vi "Single Slow IV v1.9.vi"() -> ()   [LabVIEW 2024]
uses:
  <vilib>/Utility/file.llb/Write Delimited Spreadsheet (DBL).vi
panel:
  out "Measured current":dbl=9.843554687500001e-05
  out "Current variable":dbl=8.0
  in  "stop":bool
  in  "Tab Control 2":T1(tab)
  out "cRIO data plot":cluster{"Y":dbl[], "Y":dbl[]}[](graph)=[{"Y"=[-8.0, -7.9, -7.8, -7.7, -7.6, -7.5, -7.4, -7.3, -7.2, -7.1, -7.0, -6.9, -6.8, -6.7, -6.6, -6.5, -6.4, -6.3, -6.2, -6.1, -6.0, -5.9, -5.8, -5.699999999999999, -5.6, -5.5, -5.4, -5.3, -5.199999999999999, -5.1, -5.0, -4.9, -4.8, -4.699999999999999, -4.6, -4.5, -4.4, -4.3, -4.199999999999999, -4.1, -4.0, -3.8999999999999995, -3.8, -3.7, -3.5999999999999996, -3.5, -3.3999999999999995, -3.3, -3.1999999999999993, -3.0999999999999996, -3.0, -2.8999999999999995, -2.8, -2.6999999999999993, -2.5999999999999996, -2.5, -2.3999999999999995, -2.3, -2.1999999999999993, -2.0999999999999996, -2.0, -1.8999999999999995, -1.7999999999999998, -1.6999999999999993, -1.5999999999999996, -1.5, -1.3999999999999995, -1.2999999999999998, -1.1999999999999993, -1.0999999999999996, -1.0, -0.8999999999999995, -0.7999999999999998, -0.6999999999999993, -0.5999999999999996, -0.5, -0.39999999999999947, -0.2999999999999998, -0.1999999999999993, -0.09999999999999964, 0.0, 0.09999999999999964, 0.20000000000000107, 0.3000000000000007, 0.40000000000000036, 0.5, 0.5999999999999996, 0.7000000000000011, 0.8000000000000007, 0.9000000000000004, 1.0, 1.0999999999999996, 1.200000000000001, 1.3000000000000007, 1.4000000000000004, 1.5, 1.6000000000000014, 1.700000000000001, 1.8000000000000007, 1.9000000000000004, 2.0, 2.1000000000000014, 2.200000000000001, 2.3000000000000007, 2.4000000000000004, 2.5, 2.6000000000000014, 2.700000000000001, 2.8000000000000007, 2.9000000000000004, 3.0, 3.1000000000000014, 3.200000000000001, 3.3000000000000007, 3.4000000000000004, 3.5, 3.6000000000000014, 3.700000000000001, 3.8000000000000007, 3.9000000000000004, 4.0, 4.100000000000001, 4.200000000000001, 4.300000000000001, 4.4, 4.5, 4.600000000000001, 4.700000000000001, 4.800000000000001, 4.9, 5.0, 5.100000000000001, 5.200000000000001, 5.300000000000001, 5.4, 5.5, 5.600000000000001, 5.700000000000001, 5.800000000000001, 5.9, 6.0, 6.100000000000001, 6.200000000000001, 6.300000000000001, 6.4, 6.5, 6.600000000000001, 6.700000000000001, 6.800000000000001, 6.9, 7.0, 7.100000000000001, 7.200000000000001, 7.300000000000001, 7.4, 7.5, 7.600000000000001, 7.700000000000001, 7.800000000000001, 7.9, 8.0], "Y"=[-9.206982421875e-05, -9.123583984375001e-05, -9.0050048828125e-05, -8.9024169921875e-05, -8.74638671875e-05, -8.596240234375e-05, -8.4284423828125e-05, -8.4033203125e-05, -8.22138671875e-05, -8.17998046875e-05, -7.970263671875001e-05, -7.86416015625e-05, -7.7489990234375e-05, -7.634960937500002e-05, -7.5437255859375e-05, -7.3202880859375e-05, -7.2150634765625e-05, -7.0770263671875e-05, -6.9876953125e-05, -6.917724609375e-05, -6.7115966796875e-05, -6.57978515625e-05, -6.494262695312501e-05, -6.326611328125001e-05, -6.2572265625e-05, -6.1506103515625e-05, -5.95595703125e-05, -5.860961914062501e-05, -5.706689453125e-05, -5.5826416015625e-05, -5.4549804687500006e-05, -5.3463378906250003e-05, -5.217504882812501e-05, -5.180908203125e-05, -5.023095703125e-05, -4.85771484375e-05, -4.7686279296875006e-05, -4.5836181640625006e-05, -4.574560546875e-05, -4.3756591796875e-05, -4.281591796875e-05, -4.1905761718750005e-05, -4.018115234375e-05, -3.9669921875000005e-05, -3.756884765625e-05, -3.6853759765625e-05, -3.5033203125e-05, -3.39482421875e-05, -3.3036865234375006e-05, -3.1870117187500004e-05, -3.1013671875e-05, -2.8885498046875004e-05, -2.8427490234375004e-05, -2.6702636718750003e-05, -2.4520019531250002e-05, -2.4367431640625002e-05, -2.2253173828125002e-05, -2.0526123046875003e-05, -1.94365234375e-05, -1.7531250000000003e-05, -1.506103515625e-05, -1.3855712890625e-05, -1.1485595703125001e-05, 2.761474609375e-06, 3.5068359375e-06, 3.8090820312500003e-06, 3.463134765625e-06, 3.7795410156250004e-06, 3.895263671875e-06, 3.617919921875e-06, 3.613525390625e-06, 3.5175781250000006e-06, 3.6145019531250005e-06, 3.396728515625e-06, 3.634765625e-06, 4.0371093750000005e-06, 3.047119140625e-06, 3.0192871093750003e-06, 3.9873046875e-06, 3.709716796875e-06, 4.1784667968750004e-06, 3.1230468750000003e-06, 3.239501953125e-06, 3.625732421875e-06, 3.1704101562500007e-06, 3.2299804687500005e-06, 2.862060546875e-06, 3.019775390625e-06, 3.914794921875e-06, 2.9777832031250003e-06, 3.0734863281250003e-06, 3.599609375e-06, 4.07275390625e-06, 3.518798828125e-06, 3.12060546875e-06, 3.6604003906250003e-06, 3.5278320312500003e-06, 3.673095703125e-06, 3.321044921875e-06, 3.1831054687500002e-06, 2.845947265625e-06, 3.845458984375e-06, 2.99951171875e-06, 3.86474609375e-06, 3.15380859375e-06, 3.2424316406250003e-06, 2.99609375e-06, 3.0578613281250003e-06, 3.404052734375e-06, 3.069091796875e-06, 3.40576171875e-06, 3.6384277343750003e-06, 3.1594238281250003e-06, 3.117431640625e-06, 3.7443847656250004e-06, 3.3139648437500002e-06, 4.055908203125e-06, 3.967041015625001e-06, 3.4658203125000005e-06, 3.98486328125e-06, 3.3828125e-06, 2.8564453125e-06, 2.8784179687500005e-06, 3.65771484375e-06, 3.5463867187499998e-06, 3.62353515625e-06, 2.9807128906250003e-06, 3.842041015625e-06, 2.603271484375e-06, 3.2207031249999997e-06, 6.1815673828125e-05, 6.23212890625e-05, 6.31748046875e-05, 6.61025390625e-05, 6.607885742187501e-05, 6.750683593750001e-05, 6.8930908203125e-05, 6.983105468750001e-05, 7.101293945312501e-05, 7.237768554687501e-05, 7.396655273437501e-05, 7.493896484375e-05, 7.680566406250001e-05, 7.747998046875001e-05, 7.880883789062501e-05, 8.093432617187501e-05, 8.1664794921875e-05, 8.31416015625e-05, 8.37529296875e-05, 8.49853515625e-05, 8.6370849609375e-05, 8.742211914062501e-05, 8.871997070312499e-05, 9.0783447265625e-05, 9.1563720703125e-05, 9.27861328125e-05, 9.3794189453125e-05, 9.588281250000001e-05, 9.62431640625e-05, 9.771386718750001e-05, 9.843554687500001e-05]}, {"Y"=[-8.0, -7.9, -7.8, -7.7, -7.6, -7.5, -7.4, -7.3, -7.2, -7.1, -7.0, -6.9, -6.8, -6.7, -6.6, -6.5, -6.4, -6.3, -6.2, -6.1, -6.0, -5.9, -5.8, -5.699999999999999, -5.6, -5.5, -5.4, -5.3, -5.199999999999999, -5.1, -5.0, -4.9, -4.8, -4.699999999999999, -4.6, -4.5, -4.4, -4.3, -4.199999999999999, -4.1, -4.0, -3.8999999999999995, -3.8, -3.7, -3.5999999999999996, -3.5, -3.3999999999999995, -3.3, -3.1999999999999993, -3.0999999999999996, -3.0, -2.8999999999999995, -2.8, -2.6999999999999993, -2.5999999999999996, -2.5, -2.3999999999999995, -2.3, -2.1999999999999993, -2.0999999999999996, -2.0, -1.8999999999999995, -1.7999999999999998, -1.6999999999999993, -1.5999999999999996, -1.5, -1.3999999999999995, -1.2999999999999998, -1.1999999999999993, -1.0999999999999996, -1.0, -0.8999999999999995, -0.7999999999999998, -0.6999999999999993, -0.5999999999999996, -0.5, -0.39999999999999947, -0.2999999999999998, -0.1999999999999993, -0.09999999999999964, 0.0, 0.09999999999999964, 0.20000000000000107, 0.3000000000000007, 0.40000000000000036, 0.5, 0.5999999999999996, 0.7000000000000011, 0.8000000000000007, 0.9000000000000004, 1.0, 1.0999999999999996, 1.200000000000001, 1.3000000000000007, 1.4000000000000004, 1.5, 1.6000000000000014, 1.700000000000001, 1.8000000000000007, 1.9000000000000004, 2.0, 2.1000000000000014, 2.200000000000001, 2.3000000000000007, 2.4000000000000004, 2.5, 2.6000000000000014, 2.700000000000001, 2.8000000000000007, 2.9000000000000004, 3.0, 3.1000000000000014, 3.200000000000001, 3.3000000000000007, 3.4000000000000004, 3.5, 3.6000000000000014, 3.700000000000001, 3.8000000000000007, 3.9000000000000004, 4.0, 4.100000000000001, 4.200000000000001, 4.300000000000001, 4.4, 4.5, 4.600000000000001, 4.700000000000001, 4.800000000000001, 4.9, 5.0, 5.100000000000001, 5.200000000000001, 5.300000000000001, 5.4, 5.5, 5.600000000000001, 5.700000000000001, 5.800000000000001, 5.9, 6.0, 6.100000000000001, 6.200000000000001, 6.300000000000001, 6.4, 6.5, 6.600000000000001, 6.700000000000001, 6.800000000000001, 6.9, 7.0, 7.100000000000001, 7.200000000000001, 7.300000000000001, 7.4, 7.5, 7.600000000000001, 7.700000000000001, 7.800000000000001, 7.9, 8.0], "Y"=[-7.86046142578125, -7.767216796875, -7.65550537109375, -7.5608349609375, -7.46653076171875, -7.372138671875, -7.27083251953125, -7.16314453125, -7.0821533203125, -6.9716455078125, -6.8779638671875, -6.7803369140625, -6.6772607421875, -6.58179443359375, -6.48176513671875, -6.3890576171875, -6.30079345703125, -6.1901513671875, -6.08994384765625, -5.99364501953125, -5.90613525390625, -5.80239990234375, -5.6935595703125, -5.60642822265625, -5.503076171875, -5.40948486328125, -5.31495361328125, -5.20950927734375, -5.12597412109375, -5.015322265625, -4.92371337890625, -4.8275048828125, -4.72239013671875, -4.6128369140625, -4.525625, -4.4351318359375, -4.326376953125, -4.22822509765625, -4.12566162109375, -4.04466064453125, -3.92775390625, -3.84257080078125, -3.73724365234375, -3.6371923828125, -3.547646484375, -3.44628662109375, -3.35387451171875, -3.2511572265625, -3.15429443359375, -3.0433935546875, -2.95488525390625, -2.86181396484375, -2.75966064453125, -2.65872314453125, -2.56373779296875, -2.454013671875, -2.364658203125, -2.27458740234375, -2.16810302734375, -2.069677734375, -1.98487548828125, -1.8732666015625, -1.76655517578125, -1.67587646484375, -1.5775830078125, -1.48527099609375, -1.3890234375, -1.28921142578125, -1.19949462890625, -1.09199462890625, -0.99200927734375, -0.89333984375, -0.78442138671875, -0.71025390625, -0.60267578125, -0.5152294921875, -0.4033349609375, -0.3050390625, -0.2094189453125, -0.11229736328125, -0.00902099609375, 0.08693603515625, 0.19283447265625, 0.27955078125, 0.3707275390625, 0.47876708984375, 0.58367919921875, 0.67087158203125, 0.76869384765625, 0.864560546875, 0.96866943359375, 1.064345703125, 1.16065185546875, 1.269091796875, 1.3601904296875, 1.45966064453125, 1.56078125, 1.6553076171875, 1.7527880859375, 1.85359375, 1.951552734375, 2.03806396484375, 2.14762939453125, 2.24283935546875, 2.35185791015625, 2.43536376953125, 2.5359130859375, 2.63140869140625, 2.73725341796875, 2.824853515625, 2.92412353515625, 3.027626953125, 3.13206298828125, 3.2274755859375, 3.30878173828125, 3.4181787109375, 3.511396484375, 3.61201904296875, 3.71666259765625, 3.80529296875, 3.90835205078125, 4.0163134765625, 4.10751220703125, 4.19839111328125, 4.2906494140625, 4.394130859375, 4.50539794921875, 4.58885498046875, 4.69849853515625, 4.78844482421875, 4.87513427734375, 4.997216796875, 5.1003955078125, 5.1753564453125, 5.27702880859375, 5.38421630859375, 5.4756396484375, 5.58140869140625, 5.677392578125, 5.76447021484375, 5.86692626953125, 5.976591796875, 6.055517578125, 6.17364013671875, 6.25421875, 6.344013671875, 6.46185546875, 6.54348388671875, 6.65496337890625, 6.74595947265625, 6.84517822265625, 6.94483642578125, 7.0402783203125, 7.13680908203125, 7.2312109375, 7.33786865234375, 7.4353271484375, 7.524521484375, 7.63709716796875, 7.72033447265625, 7.82843017578125]}, {"Y"=[-8.0, -7.9, -7.8, -7.7, -7.6, -7.5, -7.4, -7.3, -7.2, -7.1, -7.0, -6.9, -6.8, -6.7, -6.6, -6.5, -6.4, -6.3, -6.2, -6.1, -6.0, -5.9, -5.8, -5.699999999999999, -5.6, -5.5, -5.4, -5.3, -5.199999999999999, -5.1, -5.0, -4.9, -4.8, -4.699999999999999, -4.6, -4.5, -4.4, -4.3, -4.199999999999999, -4.1, -4.0, -3.8999999999999995, -3.8, -3.7, -3.5999999999999996, -3.5, -3.3999999999999995, -3.3, -3.1999999999999993, -3.0999999999999996, -3.0, -2.8999999999999995, -2.8, -2.6999999999999993, -2.5999999999999996, -2.5, -2.3999999999999995, -2.3, -2.1999999999999993, -2.0999999999999996, -2.0, -1.8999999999999995, -1.7999999999999998, -1.6999999999999993, -1.5999999999999996, -1.5, -1.3999999999999995, -1.2999999999999998, -1.1999999999999993, -1.0999999999999996, -1.0, -0.8999999999999995, -0.7999999999999998, -0.6999999999999993, -0.5999999999999996, -0.5, -0.39999999999999947, -0.2999999999999998, -0.1999999999999993, -0.09999999999999964, 0.0, 0.09999999999999964, 0.20000000000000107, 0.3000000000000007, 0.40000000000000036, 0.5, 0.5999999999999996, 0.7000000000000011, 0.8000000000000007, 0.9000000000000004, 1.0, 1.0999999999999996, 1.200000000000001, 1.3000000000000007, 1.4000000000000004, 1.5, 1.6000000000000014, 1.700000000000001, 1.8000000000000007, 1.9000000000000004, 2.0, 2.1000000000000014, 2.200000000000001, 2.3000000000000007, 2.4000000000000004, 2.5, 2.6000000000000014, 2.700000000000001, 2.8000000000000007, 2.9000000000000004, 3.0, 3.1000000000000014, 3.200000000000001, 3.3000000000000007, 3.4000000000000004, 3.5, 3.6000000000000014, 3.700000000000001, 3.8000000000000007, 3.9000000000000004, 4.0, 4.100000000000001, 4.200000000000001, 4.300000000000001, 4.4, 4.5, 4.600000000000001, 4.700000000000001, 4.800000000000001, 4.9, 5.0, 5.100000000000001, 5.200000000000001, 5.300000000000001, 5.4, 5.5, 5.600000000000001, 5.700000000000001, 5.800000000000001, 5.9, 6.0, 6.100000000000001, 6.200000000000001, 6.300000000000001, 6.4, 6.5, 6.600000000000001, 6.700000000000001, 6.800000000000001, 6.9, 7.0, 7.100000000000001, 7.200000000000001, 7.300000000000001, 7.4, 7.5, 7.600000000000001, 7.700000000000001, 7.800000000000001, 7.9, 8.0], "Y"=[0.0, 0.0, 0.0, 0.0, 0.0, 0.0, 0.0, 0.0, 0.0, 0.0, 0.0, 0.0, 0.0, 0.0, 0.0, 0.0, 0.0, 0.0, 0.0, 0.0, 0.0, 0.0, 0.0, 0.0, 0.0, 0.0, 0.0, 0.0, 0.0, 0.0, 0.0, 0.0, 0.0, 0.0, 0.0, 0.0, 0.0, 0.0, 0.0, 0.0, 0.0, 0.0, 0.0, 0.0, 0.0, 0.0, 0.0, 0.0, 0.0, 0.0, 0.0, 0.0, 0.0, 0.0, 0.0, 0.0, 0.0, 0.0, 0.0, 0.0, 0.0, 0.0, 0.0, 0.0, 0.0, 0.0, 0.0, 0.0, 0.0, 0.0, 0.0, 0.0, 0.0, 0.0, 0.0, 0.0, 0.0, 0.0, 0.0, 0.0, 0.0, 0.0, 0.0, 0.0, 0.0, 0.0, 0.0, 0.0, 0.0, 0.0, 0.0, 0.0, 0.0, 0.0, 0.0, 0.0, 0.0, 0.0, 0.0, 0.0, 0.0, 0.0, 0.0, 0.0, 0.0, 0.0, 0.0, 0.0, 0.0, 0.0, 0.0, 0.0, 0.0, 0.0, 0.0, 0.0, 0.0, 0.0, 0.0, 0.0, 0.0, 0.0, 0.0, 0.0, 0.0, 0.0, 0.0, 0.0, 0.0, 0.0, 0.0, 0.0, 0.0, 0.0, 0.0, 0.0, 0.0, 0.0, 0.0, 0.0, 0.0, 0.0, 0.0, 0.0, 0.0, 0.0, 0.0, 0.0, 0.0, 0.0, 0.0, 0.0, 0.0, 0.0, 0.0, 0.0, 0.0, 0.0, 0.0, 0.0, 0.0]}, {"Y"=[-8.0, -7.9, -7.8, -7.7, -7.6, -7.5, -7.4, -7.3, -7.2, -7.1, -7.0, -6.9, -6.8, -6.7, -6.6, -6.5, -6.4, -6.3, -6.2, -6.1, -6.0, -5.9, -5.8, -5.699999999999999, -5.6, -5.5, -5.4, -5.3, -5.199999999999999, -5.1, -5.0, -4.9, -4.8, -4.699999999999999, -4.6, -4.5, -4.4, -4.3, -4.199999999999999, -4.1, -4.0, -3.8999999999999995, -3.8, -3.7, -3.5999999999999996, -3.5, -3.3999999999999995, -3.3, -3.1999999999999993, -3.0999999999999996, -3.0, -2.8999999999999995, -2.8, -2.6999999999999993, -2.5999999999999996, -2.5, -2.3999999999999995, -2.3, -2.1999999999999993, -2.0999999999999996, -2.0, -1.8999999999999995, -1.7999999999999998, -1.6999999999999993, -1.5999999999999996, -1.5, -1.3999999999999995, -1.2999999999999998, -1.1999999999999993, -1.0999999999999996, -1.0, -0.8999999999999995, -0.7999999999999998, -0.6999999999999993, -0.5999999999999996, -0.5, -0.39999999999999947, -0.2999999999999998, -0.1999999999999993, -0.09999999999999964, 0.0, 0.09999999999999964, 0.20000000000000107, 0.3000000000000007, 0.40000000000000036, 0.5, 0.5999999999999996, 0.7000000000000011, 0.8000000000000007, 0.9000000000000004, 1.0, 1.0999999999999996, 1.200000000000001, 1.3000000000000007, 1.4000000000000004, 1.5, 1.6000000000000014, 1.700000000000001, 1.8000000000000007, 1.9000000000000004, 2.0, 2.1000000000000014, 2.200000000000001, 2.3000000000000007, 2.4000000000000004, 2.5, 2.6000000000000014, 2.700000000000001, 2.8000000000000007, 2.9000000000000004, 3.0, 3.1000000000000014, 3.200000000000001, 3.3000000000000007, 3.4000000000000004, 3.5, 3.6000000000000014, 3.700000000000001, 3.8000000000000007, 3.9000000000000004, 4.0, 4.100000000000001, 4.200000000000001, 4.300000000000001, 4.4, 4.5, 4.600000000000001, 4.700000000000001, 4.800000000000001, 4.9, 5.0, 5.100000000000001, 5.200000000000001, 5.300000000000001, 5.4, 5.5, 5.600000000000001, 5.700000000000001, 5.800000000000001, 5.9, 6.0, 6.100000000000001, 6.200000000000001, 6.300000000000001, 6.4, 6.5, 6.600000000000001, 6.700000000000001, 6.800000000000001, 6.9, 7.0, 7.100000000000001, 7.200000000000001, 7.300000000000001, 7.4, 7.5, 7.600000000000001, 7.700000000000001, 7.800000000000001, 7.9, 8.0], "Y"=[0.0, 0.0, 0.0, 0.0, 0.0, 0.0, 0.0, 0.0, 0.0, 0.0, 0.0, 0.0, 0.0, 0.0, 0.0, 0.0, 0.0, 0.0, 0.0, 0.0, 0.0, 0.0, 0.0, 0.0, 0.0, 0.0, 0.0, 0.0, 0.0, 0.0, 0.0, 0.0, 0.0, 0.0, 0.0, 0.0, 0.0, 0.0, 0.0, 0.0, 0.0, 0.0, 0.0, 0.0, 0.0, 0.0, 0.0, 0.0, 0.0, 0.0, 0.0, 0.0, 0.0, 0.0, 0.0, 0.0, 0.0, 0.0, 0.0, 0.0, 0.0, 0.0, 0.0, 0.0, 0.0, 0.0, 0.0, 0.0, 0.0, 0.0, 0.0, 0.0, 0.0, 0.0, 0.0, 0.0, 0.0, 0.0, 0.0, 0.0, 0.0, 0.0, 0.0, 0.0, 0.0, 0.0, 0.0, 0.0, 0.0, 0.0, 0.0, 0.0, 0.0, 0.0, 0.0, 0.0, 0.0, 0.0, 0.0, 0.0, 0.0, 0.0, 0.0, 0.0, 0.0, 0.0, 0.0, 0.0, 0.0, 0.0, 0.0, 0.0, 0.0, 0.0, 0.0, 0.0, 0.0, 0.0, 0.0, 0.0, 0.0, 0.0, 0.0, 0.0, 0.0, 0.0, 0.0, 0.0, 0.0, 0.0, 0.0, 0.0, 0.0, 0.0, 0.0, 0.0, 0.0, 0.0, 0.0, 0.0, 0.0, 0.0, 0.0, 0.0, 0.0, 0.0, 0.0, 0.0, 0.0, 0.0, 0.0, 0.0, 0.0, 0.0, 0.0, 0.0, 0.0, 0.0, 0.0, 0.0, 0.0]}]
  out "cRIO Plot 0":string="DC Voltage V"
  out "cRIO Plot 1":string="DC current uA"
  out "cRIO Plot 2":string="dV V"
  out "cRIO Plot 3":string="dI uA"
  out "Lockin X":cluster{"Y":dbl[], "Y":dbl[]}[](graph)=[{"Y"=[-8.0, -7.9, -7.8, -7.7, -7.6, -7.5, -7.4, -7.3, -7.2, -7.1, -7.0, -6.9, -6.8, -6.7, -6.6, -6.5, -6.4, -6.3, -6.2, -6.1, -6.0, -5.9, -5.8, -5.699999999999999, -5.6, -5.5, -5.4, -5.3, -5.199999999999999, -5.1, -5.0, -4.9, -4.8, -4.699999999999999, -4.6, -4.5, -4.4, -4.3, -4.199999999999999, -4.1, -4.0, -3.8999999999999995, -3.8, -3.7, -3.5999999999999996, -3.5, -3.3999999999999995, -3.3, -3.1999999999999993, -3.0999999999999996, -3.0, -2.8999999999999995, -2.8, -2.6999999999999993, -2.5999999999999996, -2.5, -2.3999999999999995, -2.3, -2.1999999999999993, -2.0999999999999996, -2.0, -1.8999999999999995, -1.7999999999999998, -1.6999999999999993, -1.5999999999999996, -1.5, -1.3999999999999995, -1.2999999999999998, -1.1999999999999993, -1.0999999999999996, -1.0, -0.8999999999999995, -0.7999999999999998, -0.6999999999999993, -0.5999999999999996, -0.5, -0.39999999999999947, -0.2999999999999998, -0.1999999999999993, -0.09999999999999964, 0.0, 0.09999999999999964, 0.20000000000000107, 0.3000000000000007, 0.40000000000000036, 0.5, 0.5999999999999996, 0.7000000000000011, 0.8000000000000007, 0.9000000000000004, 1.0, 1.0999999999999996, 1.200000000000001, 1.3000000000000007, 1.4000000000000004, 1.5, 1.6000000000000014, 1.700000000000001, 1.8000000000000007, 1.9000000000000004, 2.0, 2.1000000000000014, 2.200000000000001, 2.3000000000000007, 2.4000000000000004, 2.5, 2.6000000000000014, 2.700000000000001, 2.8000000000000007, 2.9000000000000004, 3.0, 3.1000000000000014, 3.200000000000001, 3.3000000000000007, 3.4000000000000004, 3.5, 3.6000000000000014, 3.700000000000001, 3.8000000000000007, 3.9000000000000004, 4.0, 4.100000000000001, 4.200000000000001, 4.300000000000001, 4.4, 4.5, 4.600000000000001, 4.700000000000001, 4.800000000000001, 4.9, 5.0, 5.100000000000001, 5.200000000000001, 5.300000000000001, 5.4, 5.5, 5.600000000000001, 5.700000000000001, 5.800000000000001, 5.9, 6.0, 6.100000000000001, 6.200000000000001, 6.300000000000001, 6.4, 6.5, 6.600000000000001, 6.700000000000001, 6.800000000000001, 6.9, 7.0, 7.100000000000001, 7.200000000000001, 7.300000000000001, 7.4, 7.5, 7.600000000000001, 7.700000000000001, 7.800000000000001, 7.9, 8.0], "Y"=[0.0, 0.0, 0.0, 0.0, 0.0, 0.0, 0.0, 0.0, 0.0, 0.0, 0.0, 0.0, 0.0, 0.0, 0.0, 0.0, 0.0, 0.0, 0.0, 0.0, 0.0, 0.0, 0.0, 0.0, 0.0, 0.0, 0.0, 0.0, 0.0, 0.0, 0.0, 0.0, 0.0, 0.0, 0.0, 0.0, 0.0, 0.0, 0.0, 0.0, 0.0, 0.0, 0.0, 0.0, 0.0, 0.0, 0.0, 0.0, 0.0, 0.0, 0.0, 0.0, 0.0, 0.0, 0.0, 0.0, 0.0, 0.0, 0.0, 0.0, 0.0, 0.0, 0.0, 0.0, 0.0, 0.0, 0.0, 0.0, 0.0, 0.0, 0.0, 0.0, 0.0, 0.0, 0.0, 0.0, 0.0, 0.0, 0.0, 0.0, 0.0, 0.0, 0.0, 0.0, 0.0, 0.0, 0.0, 0.0, 0.0, 0.0, 0.0, 0.0, 0.0, 0.0, 0.0, 0.0, 0.0, 0.0, 0.0, 0.0, 0.0, 0.0, 0.0, 0.0, 0.0, 0.0, 0.0, 0.0, 0.0, 0.0, 0.0, 0.0, 0.0, 0.0, 0.0, 0.0, 0.0, 0.0, 0.0, 0.0, 0.0, 0.0, 0.0, 0.0, 0.0, 0.0, 0.0, 0.0, 0.0, 0.0, 0.0, 0.0, 0.0, 0.0, 0.0, 0.0, 0.0, 0.0, 0.0, 0.0, 0.0, 0.0, 0.0, 0.0, 0.0, 0.0, 0.0, 0.0, 0.0, 0.0, 0.0, 0.0, 0.0, 0.0, 0.0, 0.0, 0.0, 0.0, 0.0, 0.0, 0.0]}, {"Y"=[-8.0, -7.9, -7.8, -7.7, -7.6, -7.5, -7.4, -7.3, -7.2, -7.1, -7.0, -6.9, -6.8, -6.7, -6.6, -6.5, -6.4, -6.3, -6.2, -6.1, -6.0, -5.9, -5.8, -5.699999999999999, -5.6, -5.5, -5.4, -5.3, -5.199999999999999, -5.1, -5.0, -4.9, -4.8, -4.699999999999999, -4.6, -4.5, -4.4, -4.3, -4.199999999999999, -4.1, -4.0, -3.8999999999999995, -3.8, -3.7, -3.5999999999999996, -3.5, -3.3999999999999995, -3.3, -3.1999999999999993, -3.0999999999999996, -3.0, -2.8999999999999995, -2.8, -2.6999999999999993, -2.5999999999999996, -2.5, -2.3999999999999995, -2.3, -2.1999999999999993, -2.0999999999999996, -2.0, -1.8999999999999995, -1.7999999999999998, -1.6999999999999993, -1.5999999999999996, -1.5, -1.3999999999999995, -1.2999999999999998, -1.1999999999999993, -1.0999999999999996, -1.0, -0.8999999999999995, -0.7999999999999998, -0.6999999999999993, -0.5999999999999996, -0.5, -0.39999999999999947, -0.2999999999999998, -0.1999999999999993, -0.09999999999999964, 0.0, 0.09999999999999964, 0.20000000000000107, 0.3000000000000007, 0.40000000000000036, 0.5, 0.5999999999999996, 0.7000000000000011, 0.8000000000000007, 0.9000000000000004, 1.0, 1.0999999999999996, 1.200000000000001, 1.3000000000000007, 1.4000000000000004, 1.5, 1.6000000000000014, 1.700000000000001, 1.8000000000000007, 1.9000000000000004, 2.0, 2.1000000000000014, 2.200000000000001, 2.3000000000000007, 2.4000000000000004, 2.5, 2.6000000000000014, 2.700000000000001, 2.8000000000000007, 2.9000000000000004, 3.0, 3.1000000000000014, 3.200000000000001, 3.3000000000000007, 3.4000000000000004, 3.5, 3.6000000000000014, 3.700000000000001, 3.8000000000000007, 3.9000000000000004, 4.0, 4.100000000000001, 4.200000000000001, 4.300000000000001, 4.4, 4.5, 4.600000000000001, 4.700000000000001, 4.800000000000001, 4.9, 5.0, 5.100000000000001, 5.200000000000001, 5.300000000000001, 5.4, 5.5, 5.600000000000001, 5.700000000000001, 5.800000000000001, 5.9, 6.0, 6.100000000000001, 6.200000000000001, 6.300000000000001, 6.4, 6.5, 6.600000000000001, 6.700000000000001, 6.800000000000001, 6.9, 7.0, 7.100000000000001, 7.200000000000001, 7.300000000000001, 7.4, 7.5, 7.600000000000001, 7.700000000000001, 7.800000000000001, 7.9, 8.0], "Y"=[0.0, 0.0, 0.0, 0.0, 0.0, 0.0, 0.0, 0.0, 0.0, 0.0, 0.0, 0.0, 0.0, 0.0, 0.0, 0.0, 0.0, 0.0, 0.0, 0.0, 0.0, 0.0, 0.0, 0.0, 0.0, 0.0, 0.0, 0.0, 0.0, 0.0, 0.0, 0.0, 0.0, 0.0, 0.0, 0.0, 0.0, 0.0, 0.0, 0.0, 0.0, 0.0, 0.0, 0.0, 0.0, 0.0, 0.0, 0.0, 0.0, 0.0, 0.0, 0.0, 0.0, 0.0, 0.0, 0.0, 0.0, 0.0, 0.0, 0.0, 0.0, 0.0, 0.0, 0.0, 0.0, 0.0, 0.0, 0.0, 0.0, 0.0, 0.0, 0.0, 0.0, 0.0, 0.0, 0.0, 0.0, 0.0, 0.0, 0.0, 0.0, 0.0, 0.0, 0.0, 0.0, 0.0, 0.0, 0.0, 0.0, 0.0, 0.0, 0.0, 0.0, 0.0, 0.0, 0.0, 0.0, 0.0, 0.0, 0.0, 0.0, 0.0, 0.0, 0.0, 0.0, 0.0, 0.0, 0.0, 0.0, 0.0, 0.0, 0.0, 0.0, 0.0, 0.0, 0.0, 0.0, 0.0, 0.0, 0.0, 0.0, 0.0, 0.0, 0.0, 0.0, 0.0, 0.0, 0.0, 0.0, 0.0, 0.0, 0.0, 0.0, 0.0, 0.0, 0.0, 0.0, 0.0, 0.0, 0.0, 0.0, 0.0, 0.0, 0.0, 0.0, 0.0, 0.0, 0.0, 0.0, 0.0, 0.0, 0.0, 0.0, 0.0, 0.0, 0.0, 0.0, 0.0, 0.0, 0.0, 0.0]}, {"Y"=[-8.0, -7.9, -7.8, -7.7, -7.6, -7.5, -7.4, -7.3, -7.2, -7.1, -7.0, -6.9, -6.8, -6.7, -6.6, -6.5, -6.4, -6.3, -6.2, -6.1, -6.0, -5.9, -5.8, -5.699999999999999, -5.6, -5.5, -5.4, -5.3, -5.199999999999999, -5.1, -5.0, -4.9, -4.8, -4.699999999999999, -4.6, -4.5, -4.4, -4.3, -4.199999999999999, -4.1, -4.0, -3.8999999999999995, -3.8, -3.7, -3.5999999999999996, -3.5, -3.3999999999999995, -3.3, -3.1999999999999993, -3.0999999999999996, -3.0, -2.8999999999999995, -2.8, -2.6999999999999993, -2.5999999999999996, -2.5, -2.3999999999999995, -2.3, -2.1999999999999993, -2.0999999999999996, -2.0, -1.8999999999999995, -1.7999999999999998, -1.6999999999999993, -1.5999999999999996, -1.5, -1.3999999999999995, -1.2999999999999998, -1.1999999999999993, -1.0999999999999996, -1.0, -0.8999999999999995, -0.7999999999999998, -0.6999999999999993, -0.5999999999999996, -0.5, -0.39999999999999947, -0.2999999999999998, -0.1999999999999993, -0.09999999999999964, 0.0, 0.09999999999999964, 0.20000000000000107, 0.3000000000000007, 0.40000000000000036, 0.5, 0.5999999999999996, 0.7000000000000011, 0.8000000000000007, 0.9000000000000004, 1.0, 1.0999999999999996, 1.200000000000001, 1.3000000000000007, 1.4000000000000004, 1.5, 1.6000000000000014, 1.700000000000001, 1.8000000000000007, 1.9000000000000004, 2.0, 2.1000000000000014, 2.200000000000001, 2.3000000000000007, 2.4000000000000004, 2.5, 2.6000000000000014, 2.700000000000001, 2.8000000000000007, 2.9000000000000004, 3.0, 3.1000000000000014, 3.200000000000001, 3.3000000000000007, 3.4000000000000004, 3.5, 3.6000000000000014, 3.700000000000001, 3.8000000000000007, 3.9000000000000004, 4.0, 4.100000000000001, 4.200000000000001, 4.300000000000001, 4.4, 4.5, 4.600000000000001, 4.700000000000001, 4.800000000000001, 4.9, 5.0, 5.100000000000001, 5.200000000000001, 5.300000000000001, 5.4, 5.5, 5.600000000000001, 5.700000000000001, 5.800000000000001, 5.9, 6.0, 6.100000000000001, 6.200000000000001, 6.300000000000001, 6.4, 6.5, 6.600000000000001, 6.700000000000001, 6.800000000000001, 6.9, 7.0, 7.100000000000001, 7.200000000000001, 7.300000000000001, 7.4, 7.5, 7.600000000000001, 7.700000000000001, 7.800000000000001, 7.9, 8.0], "Y"=[0.0, 0.0, 0.0, 0.0, 0.0, 0.0, 0.0, 0.0, 0.0, 0.0, 0.0, 0.0, 0.0, 0.0, 0.0, 0.0, 0.0, 0.0, 0.0, 0.0, 0.0, 0.0, 0.0, 0.0, 0.0, 0.0, 0.0, 0.0, 0.0, 0.0, 0.0, 0.0, 0.0, 0.0, 0.0, 0.0, 0.0, 0.0, 0.0, 0.0, 0.0, 0.0, 0.0, 0.0, 0.0, 0.0, 0.0, 0.0, 0.0, 0.0, 0.0, 0.0, 0.0, 0.0, 0.0, 0.0, 0.0, 0.0, 0.0, 0.0, 0.0, 0.0, 0.0, 0.0, 0.0, 0.0, 0.0, 0.0, 0.0, 0.0, 0.0, 0.0, 0.0, 0.0, 0.0, 0.0, 0.0, 0.0, 0.0, 0.0, 0.0, 0.0, 0.0, 0.0, 0.0, 0.0, 0.0, 0.0, 0.0, 0.0, 0.0, 0.0, 0.0, 0.0, 0.0, 0.0, 0.0, 0.0, 0.0, 0.0, 0.0, 0.0, 0.0, 0.0, 0.0, 0.0, 0.0, 0.0, 0.0, 0.0, 0.0, 0.0, 0.0, 0.0, 0.0, 0.0, 0.0, 0.0, 0.0, 0.0, 0.0, 0.0, 0.0, 0.0, 0.0, 0.0, 0.0, 0.0, 0.0, 0.0, 0.0, 0.0, 0.0, 0.0, 0.0, 0.0, 0.0, 0.0, 0.0, 0.0, 0.0, 0.0, 0.0, 0.0, 0.0, 0.0, 0.0, 0.0, 0.0, 0.0, 0.0, 0.0, 0.0, 0.0, 0.0, 0.0, 0.0, 0.0, 0.0, 0.0, 0.0]}, {"Y"=[-8.0, -7.9, -7.8, -7.7, -7.6, -7.5, -7.4, -7.3, -7.2, -7.1, -7.0, -6.9, -6.8, -6.7, -6.6, -6.5, -6.4, -6.3, -6.2, -6.1, -6.0, -5.9, -5.8, -5.699999999999999, -5.6, -5.5, -5.4, -5.3, -5.199999999999999, -5.1, -5.0, -4.9, -4.8, -4.699999999999999, -4.6, -4.5, -4.4, -4.3, -4.199999999999999, -4.1, -4.0, -3.8999999999999995, -3.8, -3.7, -3.5999999999999996, -3.5, -3.3999999999999995, -3.3, -3.1999999999999993, -3.0999999999999996, -3.0, -2.8999999999999995, -2.8, -2.6999999999999993, -2.5999999999999996, -2.5, -2.3999999999999995, -2.3, -2.1999999999999993, -2.0999999999999996, -2.0, -1.8999999999999995, -1.7999999999999998, -1.6999999999999993, -1.5999999999999996, -1.5, -1.3999999999999995, -1.2999999999999998, -1.1999999999999993, -1.0999999999999996, -1.0, -0.8999999999999995, -0.7999999999999998, -0.6999999999999993, -0.5999999999999996, -0.5, -0.39999999999999947, -0.2999999999999998, -0.1999999999999993, -0.09999999999999964, 0.0, 0.09999999999999964, 0.20000000000000107, 0.3000000000000007, 0.40000000000000036, 0.5, 0.5999999999999996, 0.7000000000000011, 0.8000000000000007, 0.9000000000000004, 1.0, 1.0999999999999996, 1.200000000000001, 1.3000000000000007, 1.4000000000000004, 1.5, 1.6000000000000014, 1.700000000000001, 1.8000000000000007, 1.9000000000000004, 2.0, 2.1000000000000014, 2.200000000000001, 2.3000000000000007, 2.4000000000000004, 2.5, 2.6000000000000014, 2.700000000000001, 2.8000000000000007, 2.9000000000000004, 3.0, 3.1000000000000014, 3.200000000000001, 3.3000000000000007, 3.4000000000000004, 3.5, 3.6000000000000014, 3.700000000000001, 3.8000000000000007, 3.9000000000000004, 4.0, 4.100000000000001, 4.200000000000001, 4.300000000000001, 4.4, 4.5, 4.600000000000001, 4.700000000000001, 4.800000000000001, 4.9, 5.0, 5.100000000000001, 5.200000000000001, 5.300000000000001, 5.4, 5.5, 5.600000000000001, 5.700000000000001, 5.800000000000001, 5.9, 6.0, 6.100000000000001, 6.200000000000001, 6.300000000000001, 6.4, 6.5, 6.600000000000001, 6.700000000000001, 6.800000000000001, 6.9, 7.0, 7.100000000000001, 7.200000000000001, 7.300000000000001, 7.4, 7.5, 7.600000000000001, 7.700000000000001, 7.800000000000001, 7.9, 8.0], "Y"=[0.0, 0.0, 0.0, 0.0, 0.0, 0.0, 0.0, 0.0, 0.0, 0.0, 0.0, 0.0, 0.0, 0.0, 0.0, 0.0, 0.0, 0.0, 0.0, 0.0, 0.0, 0.0, 0.0, 0.0, 0.0, 0.0, 0.0, 0.0, 0.0, 0.0, 0.0, 0.0, 0.0, 0.0, 0.0, 0.0, 0.0, 0.0, 0.0, 0.0, 0.0, 0.0, 0.0, 0.0, 0.0, 0.0, 0.0, 0.0, 0.0, 0.0, 0.0, 0.0, 0.0, 0.0, 0.0, 0.0, 0.0, 0.0, 0.0, 0.0, 0.0, 0.0, 0.0, 0.0, 0.0, 0.0, 0.0, 0.0, 0.0, 0.0, 0.0, 0.0, 0.0, 0.0, 0.0, 0.0, 0.0, 0.0, 0.0, 0.0, 0.0, 0.0, 0.0, 0.0, 0.0, 0.0, 0.0, 0.0, 0.0, 0.0, 0.0, 0.0, 0.0, 0.0, 0.0, 0.0, 0.0, 0.0, 0.0, 0.0, 0.0, 0.0, 0.0, 0.0, 0.0, 0.0, 0.0, 0.0, 0.0, 0.0, 0.0, 0.0, 0.0, 0.0, 0.0, 0.0, 0.0, 0.0, 0.0, 0.0, 0.0, 0.0, 0.0, 0.0, 0.0, 0.0, 0.0, 0.0, 0.0, 0.0, 0.0, 0.0, 0.0, 0.0, 0.0, 0.0, 0.0, 0.0, 0.0, 0.0, 0.0, 0.0, 0.0, 0.0, 0.0, 0.0, 0.0, 0.0, 0.0, 0.0, 0.0, 0.0, 0.0, 0.0, 0.0, 0.0, 0.0, 0.0, 0.0, 0.0, 0.0]}]
  out "Lockin Y":cluster{"Y":dbl[], "Y":dbl[]}[](graph)=[{"Y"=[-8.0, -7.9, -7.8, -7.7, -7.6, -7.5, -7.4, -7.3, -7.2, -7.1, -7.0, -6.9, -6.8, -6.7, -6.6, -6.5, -6.4, -6.3, -6.2, -6.1, -6.0, -5.9, -5.8, -5.699999999999999, -5.6, -5.5, -5.4, -5.3, -5.199999999999999, -5.1, -5.0, -4.9, -4.8, -4.699999999999999, -4.6, -4.5, -4.4, -4.3, -4.199999999999999, -4.1, -4.0, -3.8999999999999995, -3.8, -3.7, -3.5999999999999996, -3.5, -3.3999999999999995, -3.3, -3.1999999999999993, -3.0999999999999996, -3.0, -2.8999999999999995, -2.8, -2.6999999999999993, -2.5999999999999996, -2.5, -2.3999999999999995, -2.3, -2.1999999999999993, -2.0999999999999996, -2.0, -1.8999999999999995, -1.7999999999999998, -1.6999999999999993, -1.5999999999999996, -1.5, -1.3999999999999995, -1.2999999999999998, -1.1999999999999993, -1.0999999999999996, -1.0, -0.8999999999999995, -0.7999999999999998, -0.6999999999999993, -0.5999999999999996, -0.5, -0.39999999999999947, -0.2999999999999998, -0.1999999999999993, -0.09999999999999964, 0.0, 0.09999999999999964, 0.20000000000000107, 0.3000000000000007, 0.40000000000000036, 0.5, 0.5999999999999996, 0.7000000000000011, 0.8000000000000007, 0.9000000000000004, 1.0, 1.0999999999999996, 1.200000000000001, 1.3000000000000007, 1.4000000000000004, 1.5, 1.6000000000000014, 1.700000000000001, 1.8000000000000007, 1.9000000000000004, 2.0, 2.1000000000000014, 2.200000000000001, 2.3000000000000007, 2.4000000000000004, 2.5, 2.6000000000000014, 2.700000000000001, 2.8000000000000007, 2.9000000000000004, 3.0, 3.1000000000000014, 3.200000000000001, 3.3000000000000007, 3.4000000000000004, 3.5, 3.6000000000000014, 3.700000000000001, 3.8000000000000007, 3.9000000000000004, 4.0, 4.100000000000001, 4.200000000000001, 4.300000000000001, 4.4, 4.5, 4.600000000000001, 4.700000000000001, 4.800000000000001, 4.9, 5.0, 5.100000000000001, 5.200000000000001, 5.300000000000001, 5.4, 5.5, 5.600000000000001, 5.700000000000001, 5.800000000000001, 5.9, 6.0, 6.100000000000001, 6.200000000000001, 6.300000000000001, 6.4, 6.5, 6.600000000000001, 6.700000000000001, 6.800000000000001, 6.9, 7.0, 7.100000000000001, 7.200000000000001, 7.300000000000001, 7.4, 7.5, 7.600000000000001, 7.700000000000001, 7.800000000000001, 7.9, 8.0], "Y"=[0.0, 0.0, 0.0, 0.0, 0.0, 0.0, 0.0, 0.0, 0.0, 0.0, 0.0, 0.0, 0.0, 0.0, 0.0, 0.0, 0.0, 0.0, 0.0, 0.0, 0.0, 0.0, 0.0, 0.0, 0.0, 0.0, 0.0, 0.0, 0.0, 0.0, 0.0, 0.0, 0.0, 0.0, 0.0, 0.0, 0.0, 0.0, 0.0, 0.0, 0.0, 0.0, 0.0, 0.0, 0.0, 0.0, 0.0, 0.0, 0.0, 0.0, 0.0, 0.0, 0.0, 0.0, 0.0, 0.0, 0.0, 0.0, 0.0, 0.0, 0.0, 0.0, 0.0, 0.0, 0.0, 0.0, 0.0, 0.0, 0.0, 0.0, 0.0, 0.0, 0.0, 0.0, 0.0, 0.0, 0.0, 0.0, 0.0, 0.0, 0.0, 0.0, 0.0, 0.0, 0.0, 0.0, 0.0, 0.0, 0.0, 0.0, 0.0, 0.0, 0.0, 0.0, 0.0, 0.0, 0.0, 0.0, 0.0, 0.0, 0.0, 0.0, 0.0, 0.0, 0.0, 0.0, 0.0, 0.0, 0.0, 0.0, 0.0, 0.0, 0.0, 0.0, 0.0, 0.0, 0.0, 0.0, 0.0, 0.0, 0.0, 0.0, 0.0, 0.0, 0.0, 0.0, 0.0, 0.0, 0.0, 0.0, 0.0, 0.0, 0.0, 0.0, 0.0, 0.0, 0.0, 0.0, 0.0, 0.0, 0.0, 0.0, 0.0, 0.0, 0.0, 0.0, 0.0, 0.0, 0.0, 0.0, 0.0, 0.0, 0.0, 0.0, 0.0, 0.0, 0.0, 0.0, 0.0, 0.0, 0.0]}, {"Y"=[-8.0, -7.9, -7.8, -7.7, -7.6, -7.5, -7.4, -7.3, -7.2, -7.1, -7.0, -6.9, -6.8, -6.7, -6.6, -6.5, -6.4, -6.3, -6.2, -6.1, -6.0, -5.9, -5.8, -5.699999999999999, -5.6, -5.5, -5.4, -5.3, -5.199999999999999, -5.1, -5.0, -4.9, -4.8, -4.699999999999999, -4.6, -4.5, -4.4, -4.3, -4.199999999999999, -4.1, -4.0, -3.8999999999999995, -3.8, -3.7, -3.5999999999999996, -3.5, -3.3999999999999995, -3.3, -3.1999999999999993, -3.0999999999999996, -3.0, -2.8999999999999995, -2.8, -2.6999999999999993, -2.5999999999999996, -2.5, -2.3999999999999995, -2.3, -2.1999999999999993, -2.0999999999999996, -2.0, -1.8999999999999995, -1.7999999999999998, -1.6999999999999993, -1.5999999999999996, -1.5, -1.3999999999999995, -1.2999999999999998, -1.1999999999999993, -1.0999999999999996, -1.0, -0.8999999999999995, -0.7999999999999998, -0.6999999999999993, -0.5999999999999996, -0.5, -0.39999999999999947, -0.2999999999999998, -0.1999999999999993, -0.09999999999999964, 0.0, 0.09999999999999964, 0.20000000000000107, 0.3000000000000007, 0.40000000000000036, 0.5, 0.5999999999999996, 0.7000000000000011, 0.8000000000000007, 0.9000000000000004, 1.0, 1.0999999999999996, 1.200000000000001, 1.3000000000000007, 1.4000000000000004, 1.5, 1.6000000000000014, 1.700000000000001, 1.8000000000000007, 1.9000000000000004, 2.0, 2.1000000000000014, 2.200000000000001, 2.3000000000000007, 2.4000000000000004, 2.5, 2.6000000000000014, 2.700000000000001, 2.8000000000000007, 2.9000000000000004, 3.0, 3.1000000000000014, 3.200000000000001, 3.3000000000000007, 3.4000000000000004, 3.5, 3.6000000000000014, 3.700000000000001, 3.8000000000000007, 3.9000000000000004, 4.0, 4.100000000000001, 4.200000000000001, 4.300000000000001, 4.4, 4.5, 4.600000000000001, 4.700000000000001, 4.800000000000001, 4.9, 5.0, 5.100000000000001, 5.200000000000001, 5.300000000000001, 5.4, 5.5, 5.600000000000001, 5.700000000000001, 5.800000000000001, 5.9, 6.0, 6.100000000000001, 6.200000000000001, 6.300000000000001, 6.4, 6.5, 6.600000000000001, 6.700000000000001, 6.800000000000001, 6.9, 7.0, 7.100000000000001, 7.200000000000001, 7.300000000000001, 7.4, 7.5, 7.600000000000001, 7.700000000000001, 7.800000000000001, 7.9, 8.0], "Y"=[0.0, 0.0, 0.0, 0.0, 0.0, 0.0, 0.0, 0.0, 0.0, 0.0, 0.0, 0.0, 0.0, 0.0, 0.0, 0.0, 0.0, 0.0, 0.0, 0.0, 0.0, 0.0, 0.0, 0.0, 0.0, 0.0, 0.0, 0.0, 0.0, 0.0, 0.0, 0.0, 0.0, 0.0, 0.0, 0.0, 0.0, 0.0, 0.0, 0.0, 0.0, 0.0, 0.0, 0.0, 0.0, 0.0, 0.0, 0.0, 0.0, 0.0, 0.0, 0.0, 0.0, 0.0, 0.0, 0.0, 0.0, 0.0, 0.0, 0.0, 0.0, 0.0, 0.0, 0.0, 0.0, 0.0, 0.0, 0.0, 0.0, 0.0, 0.0, 0.0, 0.0, 0.0, 0.0, 0.0, 0.0, 0.0, 0.0, 0.0, 0.0, 0.0, 0.0, 0.0, 0.0, 0.0, 0.0, 0.0, 0.0, 0.0, 0.0, 0.0, 0.0, 0.0, 0.0, 0.0, 0.0, 0.0, 0.0, 0.0, 0.0, 0.0, 0.0, 0.0, 0.0, 0.0, 0.0, 0.0, 0.0, 0.0, 0.0, 0.0, 0.0, 0.0, 0.0, 0.0, 0.0, 0.0, 0.0, 0.0, 0.0, 0.0, 0.0, 0.0, 0.0, 0.0, 0.0, 0.0, 0.0, 0.0, 0.0, 0.0, 0.0, 0.0, 0.0, 0.0, 0.0, 0.0, 0.0, 0.0, 0.0, 0.0, 0.0, 0.0, 0.0, 0.0, 0.0, 0.0, 0.0, 0.0, 0.0, 0.0, 0.0, 0.0, 0.0, 0.0, 0.0, 0.0, 0.0, 0.0, 0.0]}, {"Y"=[-8.0, -7.9, -7.8, -7.7, -7.6, -7.5, -7.4, -7.3, -7.2, -7.1, -7.0, -6.9, -6.8, -6.7, -6.6, -6.5, -6.4, -6.3, -6.2, -6.1, -6.0, -5.9, -5.8, -5.699999999999999, -5.6, -5.5, -5.4, -5.3, -5.199999999999999, -5.1, -5.0, -4.9, -4.8, -4.699999999999999, -4.6, -4.5, -4.4, -4.3, -4.199999999999999, -4.1, -4.0, -3.8999999999999995, -3.8, -3.7, -3.5999999999999996, -3.5, -3.3999999999999995, -3.3, -3.1999999999999993, -3.0999999999999996, -3.0, -2.8999999999999995, -2.8, -2.6999999999999993, -2.5999999999999996, -2.5, -2.3999999999999995, -2.3, -2.1999999999999993, -2.0999999999999996, -2.0, -1.8999999999999995, -1.7999999999999998, -1.6999999999999993, -1.5999999999999996, -1.5, -1.3999999999999995, -1.2999999999999998, -1.1999999999999993, -1.0999999999999996, -1.0, -0.8999999999999995, -0.7999999999999998, -0.6999999999999993, -0.5999999999999996, -0.5, -0.39999999999999947, -0.2999999999999998, -0.1999999999999993, -0.09999999999999964, 0.0, 0.09999999999999964, 0.20000000000000107, 0.3000000000000007, 0.40000000000000036, 0.5, 0.5999999999999996, 0.7000000000000011, 0.8000000000000007, 0.9000000000000004, 1.0, 1.0999999999999996, 1.200000000000001, 1.3000000000000007, 1.4000000000000004, 1.5, 1.6000000000000014, 1.700000000000001, 1.8000000000000007, 1.9000000000000004, 2.0, 2.1000000000000014, 2.200000000000001, 2.3000000000000007, 2.4000000000000004, 2.5, 2.6000000000000014, 2.700000000000001, 2.8000000000000007, 2.9000000000000004, 3.0, 3.1000000000000014, 3.200000000000001, 3.3000000000000007, 3.4000000000000004, 3.5, 3.6000000000000014, 3.700000000000001, 3.8000000000000007, 3.9000000000000004, 4.0, 4.100000000000001, 4.200000000000001, 4.300000000000001, 4.4, 4.5, 4.600000000000001, 4.700000000000001, 4.800000000000001, 4.9, 5.0, 5.100000000000001, 5.200000000000001, 5.300000000000001, 5.4, 5.5, 5.600000000000001, 5.700000000000001, 5.800000000000001, 5.9, 6.0, 6.100000000000001, 6.200000000000001, 6.300000000000001, 6.4, 6.5, 6.600000000000001, 6.700000000000001, 6.800000000000001, 6.9, 7.0, 7.100000000000001, 7.200000000000001, 7.300000000000001, 7.4, 7.5, 7.600000000000001, 7.700000000000001, 7.800000000000001, 7.9, 8.0], "Y"=[0.0, 0.0, 0.0, 0.0, 0.0, 0.0, 0.0, 0.0, 0.0, 0.0, 0.0, 0.0, 0.0, 0.0, 0.0, 0.0, 0.0, 0.0, 0.0, 0.0, 0.0, 0.0, 0.0, 0.0, 0.0, 0.0, 0.0, 0.0, 0.0, 0.0, 0.0, 0.0, 0.0, 0.0, 0.0, 0.0, 0.0, 0.0, 0.0, 0.0, 0.0, 0.0, 0.0, 0.0, 0.0, 0.0, 0.0, 0.0, 0.0, 0.0, 0.0, 0.0, 0.0, 0.0, 0.0, 0.0, 0.0, 0.0, 0.0, 0.0, 0.0, 0.0, 0.0, 0.0, 0.0, 0.0, 0.0, 0.0, 0.0, 0.0, 0.0, 0.0, 0.0, 0.0, 0.0, 0.0, 0.0, 0.0, 0.0, 0.0, 0.0, 0.0, 0.0, 0.0, 0.0, 0.0, 0.0, 0.0, 0.0, 0.0, 0.0, 0.0, 0.0, 0.0, 0.0, 0.0, 0.0, 0.0, 0.0, 0.0, 0.0, 0.0, 0.0, 0.0, 0.0, 0.0, 0.0, 0.0, 0.0, 0.0, 0.0, 0.0, 0.0, 0.0, 0.0, 0.0, 0.0, 0.0, 0.0, 0.0, 0.0, 0.0, 0.0, 0.0, 0.0, 0.0, 0.0, 0.0, 0.0, 0.0, 0.0, 0.0, 0.0, 0.0, 0.0, 0.0, 0.0, 0.0, 0.0, 0.0, 0.0, 0.0, 0.0, 0.0, 0.0, 0.0, 0.0, 0.0, 0.0, 0.0, 0.0, 0.0, 0.0, 0.0, 0.0, 0.0, 0.0, 0.0, 0.0, 0.0, 0.0]}, {"Y"=[-8.0, -7.9, -7.8, -7.7, -7.6, -7.5, -7.4, -7.3, -7.2, -7.1, -7.0, -6.9, -6.8, -6.7, -6.6, -6.5, -6.4, -6.3, -6.2, -6.1, -6.0, -5.9, -5.8, -5.699999999999999, -5.6, -5.5, -5.4, -5.3, -5.199999999999999, -5.1, -5.0, -4.9, -4.8, -4.699999999999999, -4.6, -4.5, -4.4, -4.3, -4.199999999999999, -4.1, -4.0, -3.8999999999999995, -3.8, -3.7, -3.5999999999999996, -3.5, -3.3999999999999995, -3.3, -3.1999999999999993, -3.0999999999999996, -3.0, -2.8999999999999995, -2.8, -2.6999999999999993, -2.5999999999999996, -2.5, -2.3999999999999995, -2.3, -2.1999999999999993, -2.0999999999999996, -2.0, -1.8999999999999995, -1.7999999999999998, -1.6999999999999993, -1.5999999999999996, -1.5, -1.3999999999999995, -1.2999999999999998, -1.1999999999999993, -1.0999999999999996, -1.0, -0.8999999999999995, -0.7999999999999998, -0.6999999999999993, -0.5999999999999996, -0.5, -0.39999999999999947, -0.2999999999999998, -0.1999999999999993, -0.09999999999999964, 0.0, 0.09999999999999964, 0.20000000000000107, 0.3000000000000007, 0.40000000000000036, 0.5, 0.5999999999999996, 0.7000000000000011, 0.8000000000000007, 0.9000000000000004, 1.0, 1.0999999999999996, 1.200000000000001, 1.3000000000000007, 1.4000000000000004, 1.5, 1.6000000000000014, 1.700000000000001, 1.8000000000000007, 1.9000000000000004, 2.0, 2.1000000000000014, 2.200000000000001, 2.3000000000000007, 2.4000000000000004, 2.5, 2.6000000000000014, 2.700000000000001, 2.8000000000000007, 2.9000000000000004, 3.0, 3.1000000000000014, 3.200000000000001, 3.3000000000000007, 3.4000000000000004, 3.5, 3.6000000000000014, 3.700000000000001, 3.8000000000000007, 3.9000000000000004, 4.0, 4.100000000000001, 4.200000000000001, 4.300000000000001, 4.4, 4.5, 4.600000000000001, 4.700000000000001, 4.800000000000001, 4.9, 5.0, 5.100000000000001, 5.200000000000001, 5.300000000000001, 5.4, 5.5, 5.600000000000001, 5.700000000000001, 5.800000000000001, 5.9, 6.0, 6.100000000000001, 6.200000000000001, 6.300000000000001, 6.4, 6.5, 6.600000000000001, 6.700000000000001, 6.800000000000001, 6.9, 7.0, 7.100000000000001, 7.200000000000001, 7.300000000000001, 7.4, 7.5, 7.600000000000001, 7.700000000000001, 7.800000000000001, 7.9, 8.0], "Y"=[0.0, 0.0, 0.0, 0.0, 0.0, 0.0, 0.0, 0.0, 0.0, 0.0, 0.0, 0.0, 0.0, 0.0, 0.0, 0.0, 0.0, 0.0, 0.0, 0.0, 0.0, 0.0, 0.0, 0.0, 0.0, 0.0, 0.0, 0.0, 0.0, 0.0, 0.0, 0.0, 0.0, 0.0, 0.0, 0.0, 0.0, 0.0, 0.0, 0.0, 0.0, 0.0, 0.0, 0.0, 0.0, 0.0, 0.0, 0.0, 0.0, 0.0, 0.0, 0.0, 0.0, 0.0, 0.0, 0.0, 0.0, 0.0, 0.0, 0.0, 0.0, 0.0, 0.0, 0.0, 0.0, 0.0, 0.0, 0.0, 0.0, 0.0, 0.0, 0.0, 0.0, 0.0, 0.0, 0.0, 0.0, 0.0, 0.0, 0.0, 0.0, 0.0, 0.0, 0.0, 0.0, 0.0, 0.0, 0.0, 0.0, 0.0, 0.0, 0.0, 0.0, 0.0, 0.0, 0.0, 0.0, 0.0, 0.0, 0.0, 0.0, 0.0, 0.0, 0.0, 0.0, 0.0, 0.0, 0.0, 0.0, 0.0, 0.0, 0.0, 0.0, 0.0, 0.0, 0.0, 0.0, 0.0, 0.0, 0.0, 0.0, 0.0, 0.0, 0.0, 0.0, 0.0, 0.0, 0.0, 0.0, 0.0, 0.0, 0.0, 0.0, 0.0, 0.0, 0.0, 0.0, 0.0, 0.0, 0.0, 0.0, 0.0, 0.0, 0.0, 0.0, 0.0, 0.0, 0.0, 0.0, 0.0, 0.0, 0.0, 0.0, 0.0, 0.0, 0.0, 0.0, 0.0, 0.0, 0.0, 0.0]}]
  in  "Tab Control":T2(tab)=enum."Status"
  out "Unit":string="uA"
  in  "Tab for variable":enum32{"Current", "Magnetic field"}(tab)
  in  "Delay Time s":dbl=0.1 caption="Delay Time (s)"
  in  "AO Channel":string(combo)="AO0"
  in  "current output Scale factor":dbl=1.0
  in  "Fixed current uA":dbl=2.1
  in  "Scale factor":dbl=1.0
  in  "Field Rate mT per sec":dbl=0.1 format="%#_13g"
  in  "Magnet Device Select":string(combo)="NI DAQ Controlled V to I source"
  in  "Start":dbl=-8.0
  in  "Range":dbl=16.0
  in  "Step":dbl=0.1
  in  "Ramp type":string(combo)="Range"
  in  "Ramp up first T":bool=TRUE
  in  "x variable for plot":bool
  in  "current cRIO ch":i32
  in  "cRIO Chan 0":bool=TRUE
  in  "cRIO IP":string="//172.22.11.2"
  in  "Reading Average times":i32=100
  in  "read cRIO":bool=TRUE
  in  "Scale factor3":dbl=1.0
  in  "Channel name 3":string(combo)="dI uA"
  in  "cRIO Chan 3":bool
  in  "Scale factor2":dbl=1.0
  in  "Channel name 2":string(combo)="dV V"
  in  "cRIO Chan 2":bool
  in  "Scale factor1":dbl=1.0
  in  "Channel name 1":string(combo)="DC current uA"
  in  "cRIO Chan 1":bool=TRUE
  in  "Scale factor0":dbl=0.0001
  in  "Channel name 0":string(combo)="DC Voltage V"
  in  "Lockin address 4":string
  in  "Lockin address 3":string
  in  "Lockin address 2":string="GPIB0::9::INSTR"
  in  "Lockin address 1":string="GPIB0::8::INSTR"
  in  "Lockin 4":bool
  in  "Lockin 3":bool
  in  "Lockin 2":bool
  in  "Lockin 1":bool
  in  "Use Lockin":bool
  in  "Lockin Chan name 4":string(combo)="None"
  in  "Lockin Chan name 3":string(combo)="None"
  in  "Lockin Chan name 2":string(combo)="Current mV"
  in  "Lockin Chan name 1":string(combo)="Voltage mV"
  out "DAQ_CMD_Writer endpoint":refnum<k21>="DAQ_CMD_Writer"
  out "DAQ_AI_Reader endpoint":refnum<k21>="DAQ_AI_Reader"
  in  "Lockin and field and temperature status":string="Data File time stamp 20240118-113343\nTemperature Chan1 320.994000, Chan2 0.035014\nmagnetic field InfmT\nLockin status\n"
  in  "Temp Device":string(combo)="Elsa"
  in  "Temp Chan1":string="T5"
  in  "Temp Chan2":string="T8"
  in  "Magnetic field read device":string(combo)="None"
  in  "Record Field":bool
  out "error out":errorcluster
  in  "Contour plot folder":path=path "C:/Users/gyue/Desktop/GA01_202401"
  # "NOTE:  Tab pressed below change output signal"
  # "Voltage x factor=uA"
  # "Voltage x factor=uA"
  # "Voltage x factor=actual"
  # "cRIO channel for measured current"
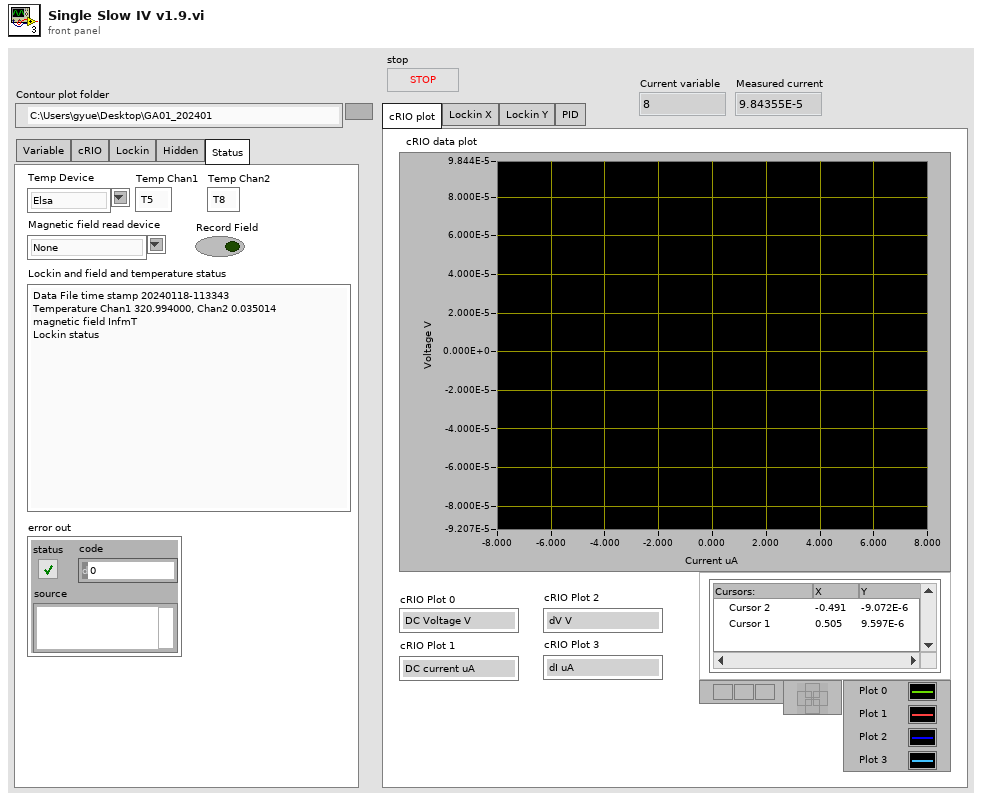
[diagram p1: front panel]
types:
  T1 = enum32{"cRIO plot", "Lockin X", "Lockin Y", "PID"}
  T2 = enum32{"Variable", "cRIO", "Lockin", "Hidden", "Status"}
  T3 = cluster{"AI0":dbl, "AI1":dbl, "AI2":dbl, "AI3":dbl}
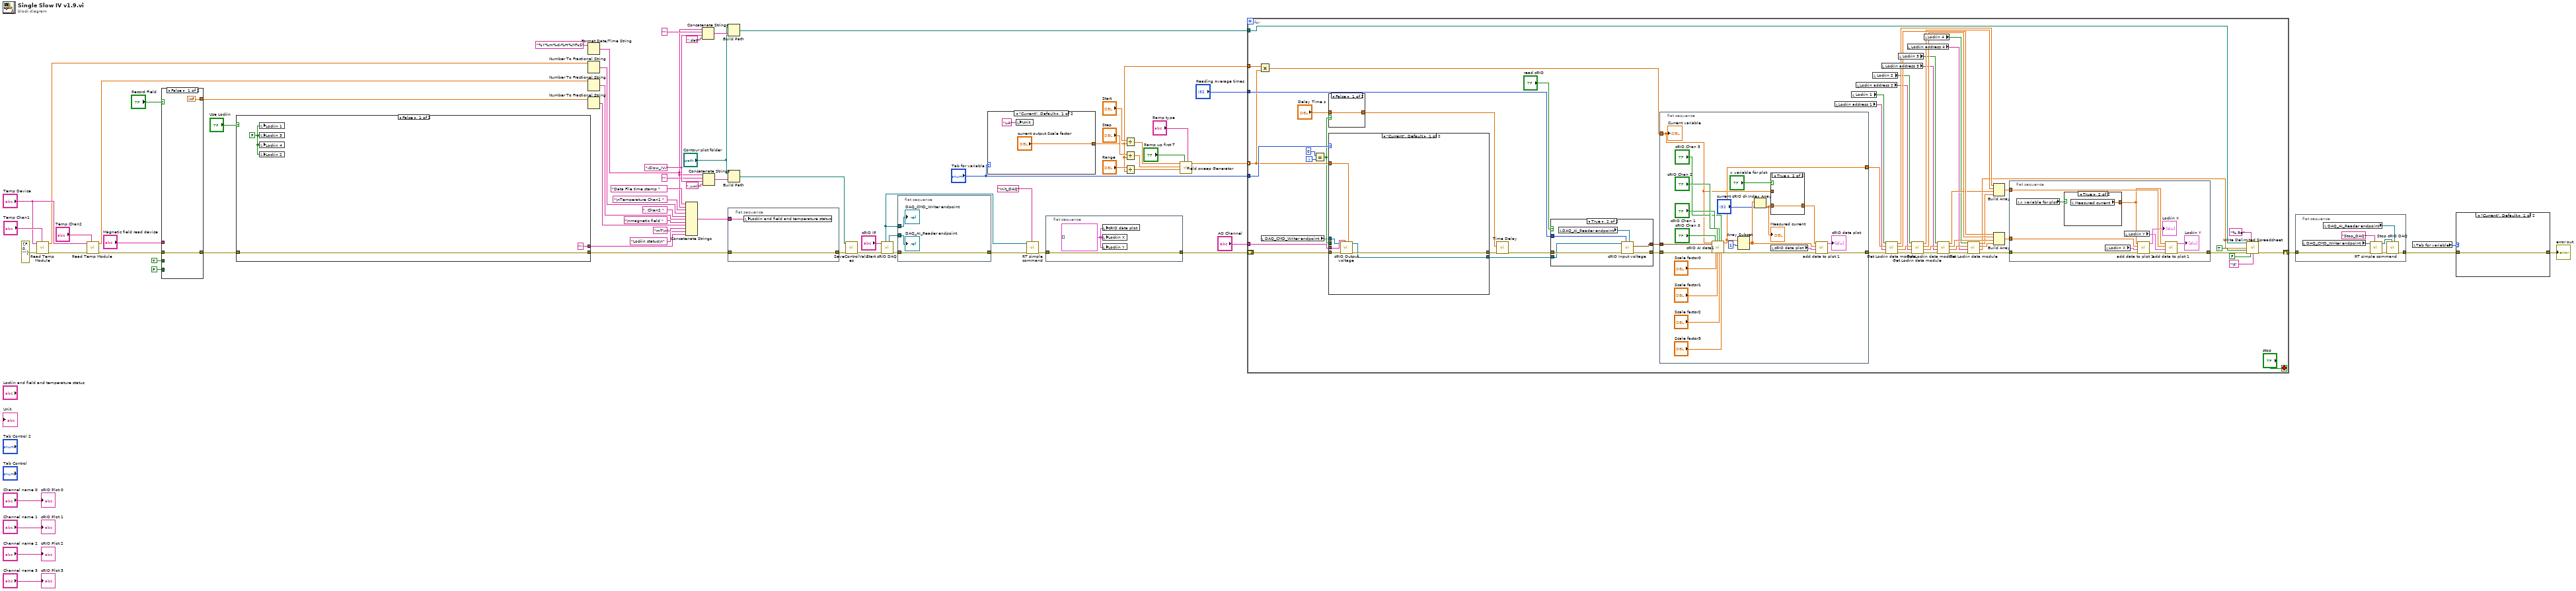
[diagram p0: block diagram]
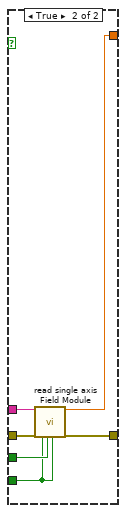
[diagram p2: hidden frame]
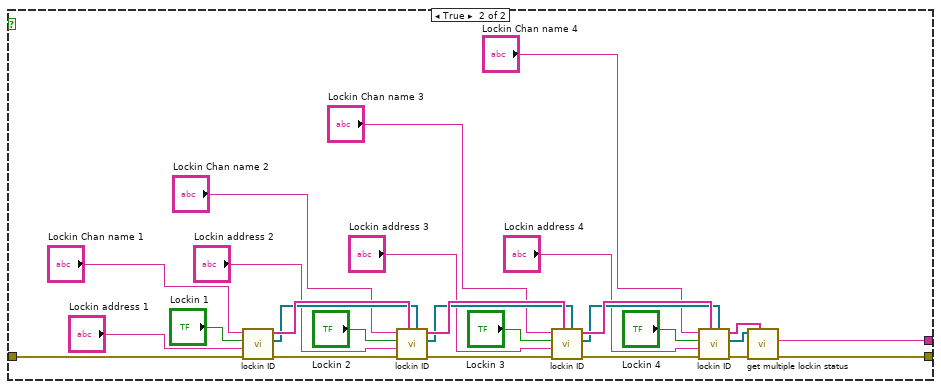
[diagram p3: hidden frame]
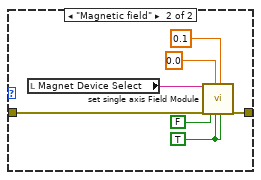
[diagram p4: hidden frame]
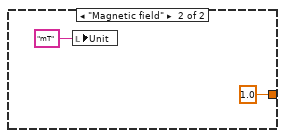
[diagram p5: hidden frame]
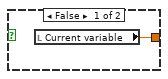
[diagram p6: hidden frame]
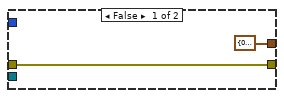
[diagram p8: hidden frame]
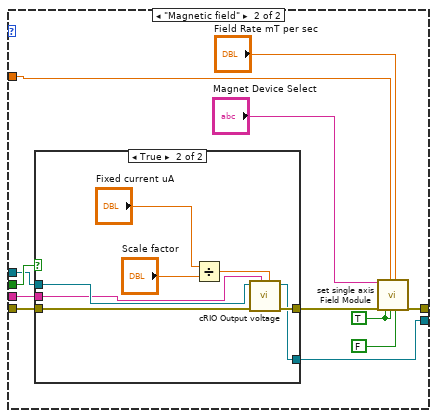
[diagram p9: hidden frame]
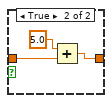
[diagram p11: hidden frame]
diagram:
  w64 = "-Slow_IV-"
  n1 = call "Read Temp Module.vi"("Temp Chan"="Temp Chan1", "error in (no error)"=errorcluster {"status"=FALSE, "code"=0, "source"=""} ("error in"), "Device"="Temp Device") -> ("error out"=w36:errorcluster, "Temperature K"=w31:dbl)  [unwired: 7 in]
  n2 = call "Read Temp Module.vi"("Temp Chan"="Temp Chan2", "error in (no error)"=w36, "Device"="Temp Device") -> ("error out"=w29:errorcluster, "Temperature K"=w30:dbl)  [unwired: 7 in]
  n3 = case shown="False" "Record Field" {
    tunnel: w29 -> [w72 w78]
    tunnel: "Magnetic field read device" -> [_ w77]
    tunnel: [inf w76] -> w27
    tunnel: TRUE ("Exec") -> [_ w75]
    tunnel: FALSE ("Init") -> [_ w74]
    tunnel: [w72 w73] -> w12
    frame False {
    }
    frame True {
      n4 = call "read single axis Field Module.vi"("Magnet Device Select"=w77, "error in (no error)"=w78, "Init"=w74, "Exec"=w75, "final"=w74) -> ("FIeld mT"=w76:dbl, "error out"=w73:errorcluster)  [unwired: 13 in]
    }
  }
  n5 = case shown="False" "Use Lockin" {
    tunnel: ["" ("Status output") w108] -> w13
    tunnel: [w81 w107] -> w11
    tunnel: w12 -> [w81 w105]
    frame False {
      w79 = FALSE ("Lockin 1")
      n6 = local write "Lockin 1"(w79) -> ()
      n7 = local write "Lockin 3"(w79) -> ()
      n8 = local write "Lockin 4"(w79) -> ()
      n9 = local write "Lockin 2"(w79) -> ()
    }
    frame True {
      n10 = call "lockin ID.vi"("error in (no error)"=w105, "Lockin address"="Lockin address 1", "Lockin on"="Lockin 1", "Lockin Chan name"="Lockin Chan name 1") -> ("error out"=w98:errorcluster, "Addresses out"=w101:refnum<visa-resource-name>[], "names out"=w102:string[])  [unwired: 5 in]
      n11 = call "lockin ID.vi"("Addresses IN"=w101, "names in"=w102, "error in (no error)"=w98, "Lockin address"="Lockin address 2", "Lockin on"="Lockin 2", "Lockin Chan name"="Lockin Chan name 2") -> ("error out"=w94:errorcluster, "Addresses out"=w95:refnum<visa-resource-name>[], "names out"=w96:string[])  [unwired: 3 in]
      n12 = call "lockin ID.vi"("Addresses IN"=w95, "names in"=w96, "error in (no error)"=w94, "Lockin address"="Lockin address 3", "Lockin on"="Lockin 3", "Lockin Chan name"="Lockin Chan name 3") -> ("error out"=w90:errorcluster, "Addresses out"=w88:refnum<visa-resource-name>[], "names out"=w89:string[])  [unwired: 3 in]
      n13 = call "lockin ID.vi"("Addresses IN"=w88, "names in"=w89, "error in (no error)"=w90, "Lockin address"="Lockin address 4", "Lockin on"="Lockin 4", "Lockin Chan name"="Lockin Chan name 4") -> ("error out"=w82:errorcluster, "Addresses out"=w83:refnum<visa-resource-name>[], "names out"=w84:string[])  [unwired: 3 in]
      n14 = call "get multiple lockin status.vi"("Device channel names"=w84, "error in (no error)"=w82, "SRS830 addresses"=w83) -> ("error out"=w107:errorcluster, "Status output"=w108:string)  [unwired: 6 in, 1 out]
    }
  }
  n15 = Format Date/Time String(time format string (%c)="%Y%m%d-%H%M%S") -> (date/time string=w23:string)  [unwired: 2 in]
  n16 = Number To Fractional String(number=w31) -> (F-format string=w20:string)  [unwired: 3 in]
  n17 = Number To Fractional String(number=w30) -> (F-format string=w19:string)  [unwired: 3 in]
  n18 = Number To Fractional String(number=w27) -> (F-format string=w17:string)  [unwired: 3 in]
  n19 = Concatenate Strings("Data File time stamp " ("string"), w23, "\nTemperature Chan1 " ("string"), w20, ", Chan2 " ("string"), w19, "\nmagnetic field " ("string"), w17, "mT\n" ("string"), "Lockin status\n" ("string"), w13) -> (w9:string)
  n20 = Concatenate Strings(w23, "" ("string"), w64, ".dat" ("string")) -> (w66:string)
  n21 = Concatenate Strings(w23, "" ("string"), w64, ".xml" ("string")) -> (w69:string)
  n22 = Build Path(base path="Contour plot folder", name or relative path=w66) -> (appended path=w51:path)
  n23 = Build Path(base path="Contour plot folder", name or relative path=w69) -> (appended path=w67:path)
  n24 = flat-sequence {
    tunnel: w11 -> [w110]
    tunnel: [w110] -> w10
    tunnel: w9 -> [w109]
    frame #0 {
      n25 = local write "Lockin and field and temperature status"(w109) -> ()
    }
  }
  n26 = call "SaveControlValues.vi"("XML File Path"=w67, "error in (no error)"=w10) -> ("error out"=w62:errorcluster)  [unwired: 8 in]
  n27 = call "Start cRIO DAQ.vi"("error in (no error)"=w62, "cRIO IP"="cRIO IP") -> ("error out"=w6:errorcluster, "DAQ_AI_Reader endpoint"=w50:refnum<k21>, "DAQ_CMD_Writer endpoint"=w3:refnum<k21>)  [unwired: 7 in]
  n28 = flat-sequence {
    tunnel: w3 -> [w113]
    tunnel: w50 -> [w112]
    tunnel: w6 -> [w111]
    tunnel: [w111] -> w5
    frame #0 {
      "DAQ_CMD_Writer endpoint" <- w113
      "DAQ_AI_Reader endpoint" <- w112
    }
  }
  n29 = case shown="\"Current\", Default" "Tab for variable" {
    tunnel: ["current output Scale factor" 1.0 ("current output Scale factor")] -> w40
    frame "Current", Default {
      n30 = local write "Unit"("uA" ("Unit")) -> ()
    }
    frame "Magnetic field" {
      n31 = local write "Unit"("mT" ("Unit")) -> ()
    }
  }
  n32 = call "RT simple command.vi"("Command"="Init_DAQ", "error in (no error)"=w5, "DAQ_CMD_Writer endpoint"=w3) -> ("error out"=w4:errorcluster)  [unwired: 7 in, 1 out]
  n33 = flat-sequence {
    tunnel: w4 -> [w119]
    tunnel: [w119] -> w7
    frame #0 {
      w118 = cluster{dbl[], dbl[]}[] [] ("appended array")
      n34 = local write "cRIO data plot"(w118) -> ()
      n35 = local write "Lockin X"(w118) -> ()
      n36 = local write "Lockin Y"(w118) -> ()
    }
  }
  n37 = Divide(x="Start", y=w40) -> (x/y=w42:dbl)
  n38 = Divide(x="Step", y=w40) -> (x/y=w55:dbl)
  n39 = Divide(x="Range", y=w40) -> (x/y=w54:dbl)
  n40 = call "Field sweep Generator.vi"("Ramp type"="Ramp type", "Ramp up first T"="Ramp up first T", "Field Radius"=w54, "Field step"=w55, "Field Origin"=w42) -> ("output array"=w52:dbl[])  [unwired: 6 in]
  n41 = for {
    tunnel: "AO Channel" -> [w159]
    tunnel: w52 -> [w160] mode=indexing
    tunnel: w51 -> [w174]
    tunnel: "Reading Average times" -> [w167]
    tunnel: "Tab for variable" -> [w161]
    tunnel: w40 -> [w155]
    shift-right: [w168] -> w1
    shift-left: w7 -> [w153]
    i -> [w165]
    stop <- "stop" stop-if-true
    n42 = Multiply(x=w155, y=w160) -> (x*y=w151:dbl)
    n43 = local read "DAQ_CMD_Writer endpoint"() -> (w120:refnum<k21>)
    n44 = Equal?(x=0, y=w165) -> (x = y?=w156:bool)
    n45 = case shown="False" w156 {
      tunnel: "Delay Time s" -> [w248 w249]
      tunnel: [w248 w251] -> w162
      frame False {
      }
      frame True {
        n46 = Add(x=5.0 ("Delay Time s"), y=w249) -> (x+y=w251:dbl)
      }
    }
    n47 = case shown="\"Current\", Default" w161 {
      tunnel: w160 -> [w225 w229]
      tunnel: w159 -> [w224 w233]
      tunnel: w153 -> [w223 w236]
      tunnel: w120 -> [w222 w235]
      tunnel: [w221 w231] -> w158
      tunnel: [w220 w234] -> w157
      tunnel: w156 -> [_ w237]
      frame "Current", Default {
        n48 = call "cRIO Output voltage.vi"("Voltage"=w225, "AO Channel"=w224, "error in (no error)"=w223, "DAQ_CMD_Writer endpoint"=w222) -> ("error out"=w221:errorcluster, "DAQ_CMD_Writer endpoint out"=w220:refnum<k21>)  [unwired: 6 in]
      }
      frame "Magnetic field" {
        w227 = TRUE ("Init")
        n49 = case shown="True" w237 {
          tunnel: w236 -> [w238 w247]
          tunnel: [w238 w246] -> w232
          tunnel: w235 -> [w239 w245]
          tunnel: [w239 w244] -> w234
          tunnel: w233 -> [_ w243]
          frame False {
          }
          frame True {
            n50 = Divide(x="Fixed current uA", y="Scale factor") -> (x/y=w241:dbl)
            n51 = call "cRIO Output voltage.vi"("Voltage"=w241, "AO Channel"=w243, "error in (no error)"=w247, "DAQ_CMD_Writer endpoint"=w245) -> ("error out"=w246:errorcluster, "DAQ_CMD_Writer endpoint out"=w244:refnum<k21>)  [unwired: 6 in]
          }
        }
        n52 = call "set single axis Field Module.vi"("Field Device Select"="Magnet Device Select", "error in (no error)"=w232, "Init"=w227, "Field Target mT or dBm"=w229, "Exec"=w227, "Field Rate mT per sec"="Field Rate mT per sec", "final"=FALSE ("Exec")) -> ("error out"=w231:errorcluster)  [unwired: 12 in]
      }
    }
    n53 = call "Time Delay"("error in (no error)"=w158, "Delay Time (s)"=w162) -> ("error out"=w170:errorcluster)  [unwired: 9 in]
    n54 = case shown="True" "read cRIO" {
      tunnel: w170 -> [w213 w219]
      tunnel: [w213 w218] -> w149
      tunnel: w167 -> [_ w217]
      tunnel: w157 -> [_ w216]
      tunnel: [T3 {"AI0"=0.0, "AI1"=0.0, "AI2"=0.0, "AI3"=0.0} ("output cluster") w215] -> w150
      frame False {
      }
      frame True {
        n55 = local read "DAQ_AI_Reader endpoint"() -> (w214:refnum<k21>)
        n56 = call "cRIO Input voltage.vi"("DAQ_AI_Reader endpoint"=w214, "Average"=w217, "error in (no error)"=w219, "DAQ_CMD_Writer endpoint"=w216) -> ("error out"=w218:errorcluster, "output cluster"=w215:T3)  [unwired: 5 in, 1 out]
      }
    }
    n57 = flat-sequence {
      tunnel: w151 -> [w190]
      tunnel: w150 -> [w208]
      tunnel: w149 -> [w207]
      tunnel: [w200] -> w148
      tunnel: [w195] -> w147
      frame #0 {
        n58 = call "cRIO AI data1.vi"("I"=w190, "Input cluster"=w208, "error in (no error)"=w207, "Chan 0"="cRIO Chan 0", "Scale factor0"="Scale factor0", "Chan 1"="cRIO Chan 1", "Scale factor1"="Scale factor1", "Chan 2"="cRIO Chan 2", "Scale factor2"="Scale factor2", "Chan 3"="cRIO Chan 3", "Scale factor3"="Scale factor3") -> ("Output data"=w195:dbl[], "error out"=w201:errorcluster)  [unwired: 7 in]
        n59 = Array Subset(array=w195, index=1) -> (w193:dbl[])  [unwired: 1 in]
        n60 = Index Array(array=w193, index="current cRIO ch") -> (element=w188:dbl)
        "Measured current" <- w188
        n61 = case shown="True" "x variable for plot" {
          tunnel: w190 -> [w210 _]
          tunnel: [w210 w211] -> w189
          tunnel: w188 -> [_ w211]
          frame False {
          }
          frame True {
          }
        }
        n62 = local read "cRIO data plot"() -> (w209:cluster{"Y":dbl[], "Y":dbl[]}[])
        n63 = call "add data to plot 1.vi"("error in (no error)"=w201, "Input graph"=w209, "Input Y array"=w193, "x"=w189) -> ("error in (no error) 2"=w200:errorcluster, "Output graph"=→"cRIO data plot":cluster{dbl[], dbl[]}[])  [unwired: 6 in]
        "Current variable" <- w190
      }
    }
    n64 = local read "Lockin address 1"() -> (w141:string)
    n65 = local read "Lockin 1"() -> (w152:bool)
    n66 = local read "Lockin address 2"() -> (w138:string)
    n67 = local read "Lockin 2"() -> (w140:bool)
    n68 = local read "Lockin address 3"() -> (w131:string)
    n69 = call "Get Lockin data module.vi"("error in (no error)"=w148, "Lockin address 1"=w141, "Output data in"=w147, "Lockin 1"=w152) -> ("error out"=w137:errorcluster, "Output data out"=w139:dbl[], "X mV"=w145:dbl, "Y mV"=w143:dbl)  [unwired: 4 in]
    n70 = local read "Lockin 3"() -> (w134:bool)
    n71 = local read "Lockin address 4"() -> (w125:string)
    n72 = call "Get Lockin data module.vi"("error in (no error)"=w137, "Lockin address 1"=w138, "Output data in"=w139, "Lockin 1"=w140) -> ("error out"=w132:errorcluster, "Output data out"=w133:dbl[], "X mV"=w135:dbl, "Y mV"=w136:dbl)  [unwired: 4 in]
    n73 = local read "Lockin 4"() -> (w128:bool)
    n74 = call "Get Lockin data module.vi"("error in (no error)"=w132, "Lockin address 1"=w131, "Output data in"=w133, "Lockin 1"=w134) -> ("error out"=w126:errorcluster, "Output data out"=w127:dbl[], "X mV"=w129:dbl, "Y mV"=w130:dbl)  [unwired: 4 in]
    n75 = call "Get Lockin data module.vi"("error in (no error)"=w126, "Lockin address 1"=w125, "Output data in"=w127, "Lockin 1"=w128) -> ("error out"=w122:errorcluster, "Output data out"=w121:dbl[], "X mV"=w123:dbl, "Y mV"=w124:dbl)  [unwired: 4 in]
    n76 = Build Array(w143, w136, w130, w124) -> (w142:dbl[])
    n77 = Build Array(w145, w135, w129, w123) -> (w144:dbl[])
    n78 = flat-sequence {
      tunnel: w122 -> [w182]
      tunnel: [w180] -> w146
      tunnel: w144 -> [w183]
      tunnel: w142 -> [w177]
      frame #0 {
        n79 = local read "x variable for plot"() -> (w176:bool)
        n80 = case shown="True" w176 {
          tunnel: [w186 w187] -> w175
          frame False {
            n81 = local read "Current variable"() -> (w186:dbl)
          }
          frame True {
            n82 = local read "Measured current"() -> (w187:dbl)
          }
        }
        n83 = local read "Lockin X"() -> (w185:cluster{"Y":dbl[], "Y":dbl[]}[])
        n84 = local read "Lockin Y"() -> (w179:cluster{"Y":dbl[], "Y":dbl[]}[])
        n85 = call "add data to plot 1.vi"("error in (no error)"=w182, "Input graph"=w185, "Input Y array"=w183, "x"=w175) -> ("error in (no error) 2"=w181:errorcluster, "Output graph"=→"Lockin X":cluster{dbl[], dbl[]}[])  [unwired: 6 in]
        n86 = call "add data to plot 1.vi"("error in (no error)"=w181, "Input graph"=w179, "Input Y array"=w177, "x"=w175) -> ("error in (no error) 2"=w180:errorcluster, "Output graph"=→"Lockin Y":cluster{dbl[], dbl[]}[])  [unwired: 6 in]
      }
    }
    n87 = call-poly <vilib>:"Write Delimited Spreadsheet.vi"("file path (dialog if empty)"=w174, "format (%.3f)"="%.9e", "1D data"=w121, "append to file? (new file:F)"=TRUE, "error in (no error)"=w146, "transpose? (no:F)"=FALSE, "delimiter (\\t)"="\t" ("delimiter (\\t)")) -> ("error out"=w168:errorcluster)  [unwired: 7 in, 1 out]
  }
  n88 = flat-sequence {
    tunnel: [w258] -> w38
    tunnel: w1 -> [w253]
    frame #0 {
      n89 = local read "DAQ_CMD_Writer endpoint"() -> (w254:refnum<k21>)
      n90 = local read "DAQ_AI_Reader endpoint"() -> (w257:refnum<k21>)
      n91 = call "RT simple command.vi"("Command"="Stop_DAQ", "error in (no error)"=w253, "DAQ_CMD_Writer endpoint"=w254) -> ("error out"=w252:errorcluster, "DAQ_CMD_Writer endpoint out"=w255:refnum<k21>)  [unwired: 7 in]
      n92 = call "Stop cRIO DAQ.vi"("DAQ_AI_Reader endpoint"=w257, "DAQ_CMD_Writer endpoint"=w255, "error in (no error)"=w252) -> ("error out"=w258:errorcluster)  [unwired: 8 in]
    }
  }
  n93 = local read "Tab for variable"() -> (w39:enum32{"Current", "Magnetic field"})
  n94 = case shown="\"Current\", Default" w39 {
    tunnel: w38 -> [w259 w263]
    tunnel: [w259 w262] -> w37
    frame "Current", Default {
    }
    frame "Magnetic field" {
      w260 = TRUE ("Exec")
      n95 = local read "Magnet Device Select"() -> (w266:string)
      n96 = call "set single axis Field Module.vi"("Field Device Select"=w266, "error in (no error)"=w263, "Init"=FALSE, "Field Target mT or dBm"=0.0 ("Field Target mT"), "Exec"=w260, "Field Rate mT per sec"=0.1, "final"=w260) -> ("error out"=w262:errorcluster)  [unwired: 12 in]
    }
  }
  "error out" <- w37
  "cRIO Plot 0" <- "Channel name 0"
  "cRIO Plot 1" <- "Channel name 1"
  "cRIO Plot 2" <- "Channel name 2"
  "cRIO Plot 3" <- "Channel name 3"
